vi "Pneumatic_Sensor_Loop.vi"(4 "Priority":i32=100, 6 "Period":i64=20, 7 "Solenoid Configuration":T5, 9 "DigitalInputDevRef":T1, 10 "AIDeviceRef":T3, 11 "Cluster":T8) -> ()   [LabVIEW 2016]
doc: "Help by FRC Team 836 - The RoboBees\n\nThis VI configures the sensors for the pneumatics."
uses:
  <userlib>/836-Libraries/Pneumatics/Support_Code/Pneumatic_Sensor_Loop.ctl
  <userlib>/836-Libraries/Pneumatics/Support_Code/Pneumatics_Status.ctl
  <vilib>/Rock Robotics/WPI/Solenoid/WPI_SolenoidValue.ctl
  <userlib>/836-Libraries/Pneumatics/Support_Code/Solenoid_Configure.ctl
  <userlib>/836-Libraries/Pneumatics/Support_Code/Pneumatics_Configuration.ctl
  <userlib>/836-Libraries/Pneumatics/Support_Code/Feedback_Method.ctl
  <vilib>/Rock Robotics/WPI/AnalogChannel/WPI_AnalogChannelDevRef.ctl
  <vilib>/Rock Robotics/SystemInterfaces/AI/FPGA_AIChannel.ctl
  <vilib>/Rock Robotics/WPI/DigitalInput/WPI_DigitalInputDevRef.ctl
  <vilib>/Rock Robotics/SystemInterfaces/DIO/FPGA_DIOChannel.ctl
  <vilib>/Platform/TimedLoop/XDataNode/timing_clust.ctl
  <vilib>/Platform/TimedLoop/XDataNode/nitl_modes.ctl
  <vilib>/Platform/TimedLoop/XDataNode/wakeup.ctl
  <vilib>/platform/TimedLoop/XDataNode/XDataNode.xnode
  <vilib>/Platform/TimedLoop/XDataNode/XDNodeRunTimeDep.lvlib
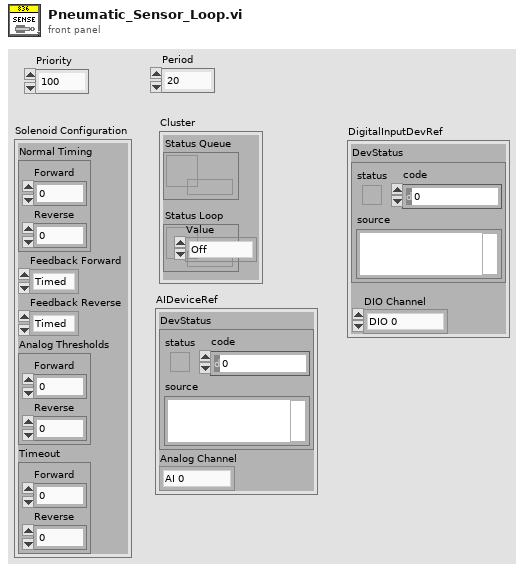
[diagram p1: front panel]
types:
  T1 = typedef "WPI_DigitalInputDevRef.ctl" = cluster{"DevStatus":errorcluster, "DIO Channel":T2}
  T2 = typedef "FPGA_DIOChannel.ctl" = enum8{"DIO 0", "DIO 1", "DIO 2", "DIO 3", "DIO 4", "DIO 5", "DIO 6", "DIO 7", "DIO 8", "DIO 9", "DIO MXP 0", "DIO MXP 1", "DIO MXP 2", "DIO MXP 3", "DIO MXP 4", "DIO MXP 5", "DIO MXP 6", "DIO MXP 7", "DIO MXP 8", "DIO MXP 9", "DIO MXP 10", "DIO MXP 11", "DIO MXP 12", "DIO MXP 13", "DIO MXP 14", "DIO MXP 15", "SPI Port CS1", "SPI Port CS2", "SPI Port CS3", "SPI Port MISO", "SPI Port MOSI", "Invalid"}
  T3 = typedef "WPI_AnalogChannelDevRef.ctl" = cluster{"DevStatus":errorcluster, "Analog Channel":T4}
  T4 = typedef "FPGA_AIChannel.ctl" = enum8{"AI 0", "AI 1", "AI 2", "AI 3", "AI MXP 0", "AI MXP 1", "AI MXP 2", "AI MXP 3", "Invalid"}
  T5 = typedef "Solenoid_Configure.ctl" = cluster{"Normal Timing":T6, "Feedback Forward":T7, "Feedback Reverse":T7, "Analog Thresholds":T6, "Timeout":T6}
  T6 = typedef "Pneumatics_Configuration.ctl" = cluster{"Forward":dbl, "Reverse":dbl}
  T7 = typedef "Feedback_Method.ctl" = enum16{"Timed", "Analog", "Digital", "Analog (Inverted)", "Digital (Inverted)"}
  T8 = typedef "Pneumatic_Sensor_Loop.ctl" = cluster{"Status Queue":refnum<queue>, "Status Loop":refnum<k33>, "Relay Value":T9}
  T9 = typedef "WPI_SolenoidValue.ctl" = enum16{"Off", "On", "Forward", "Reverse"}
  T10 = typedef "Pneumatics_Status.ctl" = enum16{"Forward", "Reverse", "Moving"}
  T11 = typedef "XDNodeRunTimeDep.lvlib/timing_clust.ctl" = cluster{"Expected End [f-1]":u64, "Actual End [f-1]":u64, "Finished Late? [f-1]":bool, "Expected End [i-1]":u64, "Actual End [i-1]":u64, "Finished Late? [i-1]":bool, "Expected Start [i]":u64, "Actual Start [i]":u64, "Expected Start [f]":u64, "Actual Start [f]":u64, "Source Name":string, "Structure Name":string, "Period":i64, "Deadline":i64, "Offset":i64, "Start":i64, "Priority":i32, "Timeout":i32, "Mode":T12, "Wakeup Reason":T13, "Error":errorcluster, "Source Type":string, "Secondary Source Type":string, "Global End Time":u64, "Global Start Time":u64, "Frame Duration":u64, "Iteration Duration":u64, "Assigned CPU":i32, "I/O Scan Engine Mode":u32}
  T12 = typedef "XDNodeRunTimeDep.lvlib/nitl_modes.ctl" = enum32{"No Change", "Process missed periods, maintain original phase", "Discard missed periods, maintain original phase", "Process missed periods, ignore original phase", "Discard missed periods, ignore original phase"}
  T13 = typedef "XDNodeRunTimeDep.lvlib/wakeup.ctl" = enum32{"Normal", "Aborted", "Asynchronous wakeup", "Timing source error", "Timed loop error", "Timeout"}
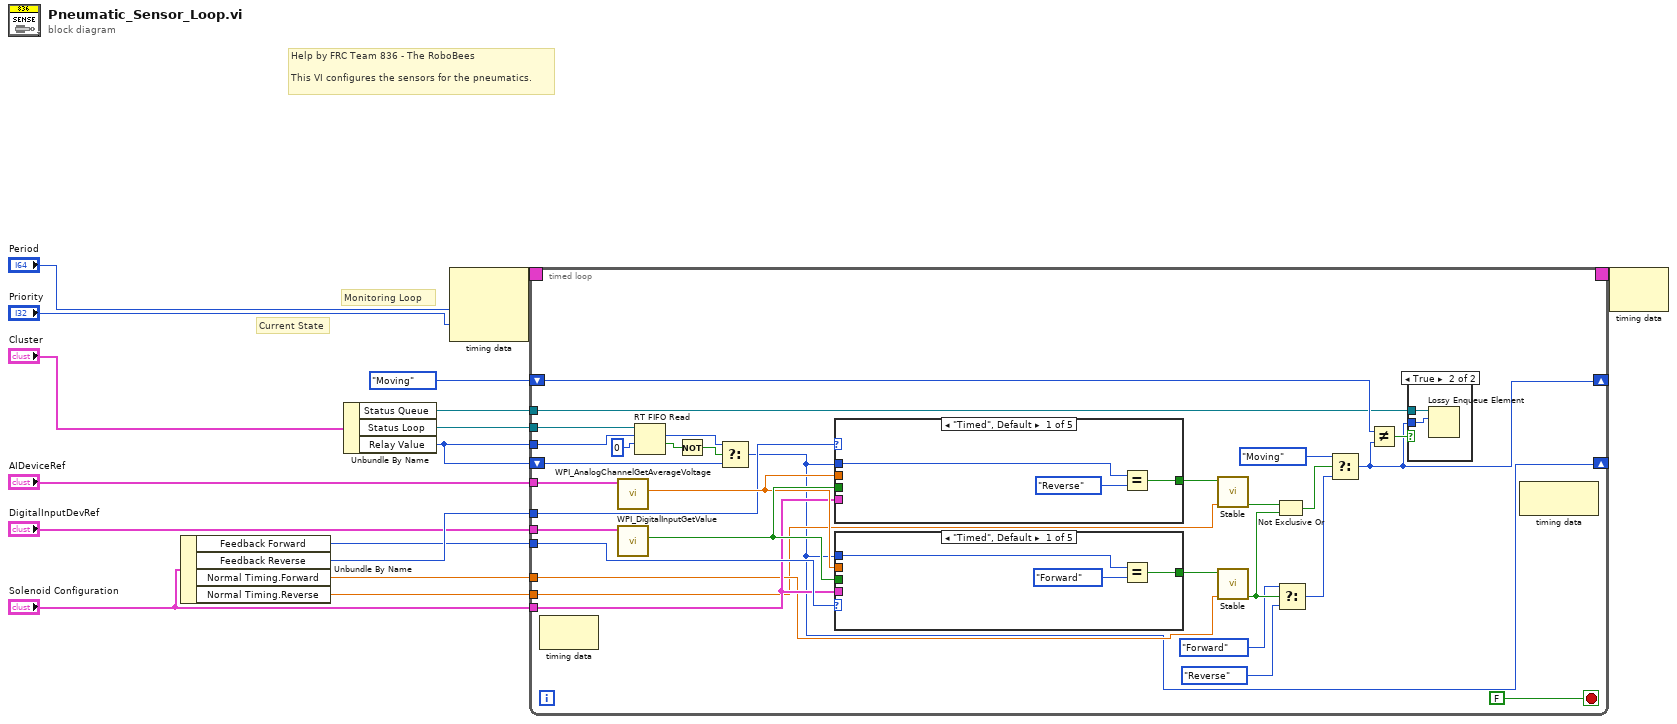
[diagram p0: block diagram]
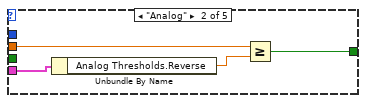
[diagram p3: hidden frame]
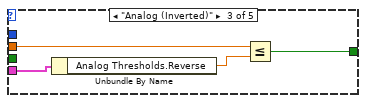
[diagram p4: hidden frame]
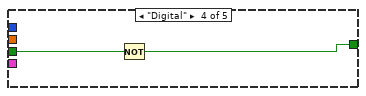
[diagram p5: hidden frame]
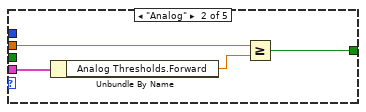
[diagram p7: hidden frame]
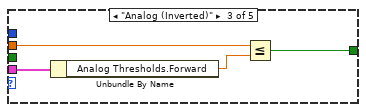
[diagram p8: hidden frame]
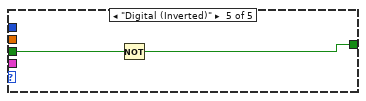
[diagram p10: hidden frame]
diagram:
  # "Help by FRC Team 836 - The RoboBees\n\nThis VI configures the sensors for the pneumatics."
  # "Monitoring Loop"
  # "Current State"
  n1 = Unbundle By Name("Solenoid Configuration") -> ("Feedback Forward"=w6:T7, "Feedback Reverse"=w7:T7, "Normal Timing.Forward"=w9:dbl, "Normal Timing.Reverse"=w10:dbl)
  n2 = Unbundle By Name("Cluster") -> ("Status Queue"=w12:refnum<queue>, "Status Loop"=w13:refnum<k33>, "Relay Value"=w14:T9)
  n3 = node-c288("Period", "Priority") -> (w16:T11)  [unwired: 1 in]
  n4 = timed-loop {
    timing: w16 -> [_]
    timing-out: [_] -> w15
    tunnel: "DigitalInputDevRef" -> [w46]
    tunnel: "AIDeviceRef" -> [w45]
    tunnel: w6 -> [w44]
    tunnel: w7 -> [w38]
    tunnel: "Solenoid Configuration" -> [w40]
    shift-right: [w28] -> _
    shift-left: Pneumatics_Status."Moving" ("Enum") -> [w30]
    tunnel: w13 -> [w24]
    tunnel: w12 -> [w25]
    tunnel: w9 -> [w27]
    tunnel: w10 -> [w26]
    shift-right: [w19] -> _
    shift-left: w14 -> [w18]
    tunnel: w14 -> [w17]
    stop <- FALSE stop-if-true
    n5 = node-c288() -> ()  [unwired: 1 in, 1 out]
    n6 = call <vilib>:"WPI_AnalogChannelGetAverageVoltage.vi"("AIDeviceRef"=w45) -> ("Voltage"=w41:dbl)  [unwired: 8 in, 2 out]
    n7 = call <vilib>:"WPI_DigitalInputGetValue.vi"("DigitalInputDevRef"=w46) -> ("Value"=w42:bool)  [unwired: 8 in, 2 out]
    n8 = RT FIFO Read(0:w24, 1:w17, 2:0 ("timeout in ms (-1)")) -> (9:w20:T9, 10:w22:bool)  [unwired: 1 in, 3 out]
    n9 = Not(x=w22) -> (.not. x?=w21:bool)
    n10 = Select(t=w20, s=w21, f=w18) -> (s? t:f=w19:T9)
    n11 = case shown="\"Timed\", Default" w38 {
      tunnel: w42 -> [_ _ _ w62 w63]
      tunnel: [w52 w55 w59 w61 w63] -> w39
      tunnel: w41 -> [_ w56 w60 _ _]
      tunnel: w40 -> [_ w54 w58 _ _]
      tunnel: w19 -> [w51 _ _ _ _]
      frame "Timed", Default {
        n12 = Equal?(x=w51, y=WPI_SolenoidValue."Reverse") -> (x = y?=w52:bool)
      }
      frame "Analog" {
        n13 = Unbundle By Name(w54) -> ("Analog Thresholds.Reverse"=w53:dbl)
        n14 = Greater Or Equal?(x=w56, y=w53) -> (x >= y?=w55:bool)
      }
      frame "Analog (Inverted)" {
        n15 = Unbundle By Name(w58) -> ("Analog Thresholds.Reverse"=w57:dbl)
        n16 = Less Or Equal?(x=w60, y=w57) -> (x <= y?=w59:bool)
      }
      frame "Digital" {
        n17 = Not(x=w62) -> (.not. x?=w61:bool)
      }
      frame "Digital (Inverted)" {
      }
    }
    n18 = case shown="\"Timed\", Default" w44 {
      tunnel: w42 -> [_ _ _ w75 w77]
      tunnel: [w66 w69 w73 w75 w76] -> w43
      tunnel: w41 -> [_ w70 w74 _ _]
      tunnel: w40 -> [_ w68 w72 _ _]
      tunnel: w19 -> [w65 _ _ _ _]
      frame "Timed", Default {
        n19 = Equal?(x=w65, y=WPI_SolenoidValue."Forward") -> (x = y?=w66:bool)
      }
      frame "Analog" {
        n20 = Unbundle By Name(w68) -> ("Analog Thresholds.Forward"=w67:dbl)
        n21 = Greater Or Equal?(x=w70, y=w67) -> (x >= y?=w69:bool)
      }
      frame "Analog (Inverted)" {
        n22 = Unbundle By Name(w72) -> ("Analog Thresholds.Forward"=w71:dbl)
        n23 = Less Or Equal?(x=w74, y=w71) -> (x <= y?=w73:bool)
      }
      frame "Digital" {
      }
      frame "Digital (Inverted)" {
        n24 = Not(x=w77) -> (.not. x?=w76:bool)
      }
    }
    n25 = call <userlib>:"Stable.vi"("Eval Period (sec)"=w26, "Signal Input"=w39) -> ("Stable"=w37:bool)  [unwired: 9 in]
    n26 = call <userlib>:"Stable.vi"("Eval Period (sec)"=w27, "Signal Input"=w43) -> ("Stable"=w34:bool)  [unwired: 9 in]
    n27 = Not Exclusive Or(1:w34, 2:w37) -> (0:w35:bool)
    n28 = Select(t=Pneumatics_Status."Forward" ("Enum"), s=w34, f=Pneumatics_Status."Reverse" ("Enum")) -> (s? t:f=w31:T10)
    n29 = Select(t=Pneumatics_Status."Moving" ("Enum"), s=w35, f=w31) -> (s? t:f=w28:T10)
    n30 = Not Equal?(x=w30, y=w28) -> (x != y?=w29:bool)
    n31 = case shown="True" w29 {
      tunnel: w28 -> [_ w48]
      tunnel: w25 -> [_ w49]
      frame False {
      }
      frame True {
        n32 = Lossy Enqueue Element(queue=w49, element=w48) -> ()  [unwired: 1 in, 4 out]
      }
    }
    n33 = node-c288() -> ()  [unwired: 1 in, 1 out]
  }
  n34 = node-c288(w15) -> ()  [unwired: 1 out]
